vi "Buffered Stream to Tab-Delimited Text File.vi"() -> ()   [LabVIEW 2023]
doc: "Demonstrates the use of File I/O and Array functions to stream data to a tab-delimited text file. This example manages memory in an efficient manner to stream data to the text file at a high rate."
panel:
  out "Streaming Rate (MB/sec)":dbl
  # "Overview: Demonstrates the use of File I/O and Array functions to stream data to a tab-delimited text file. This example manages memory in an efficient manner to stream data to the text file at a high rate.\nInstructions:\n1. Run this VI, which streams data to a tab-delimited text file for 1 second.\n2. Open the [LabVIEW Data]\\Example Streamed Spreadsheet Data.txt file in a spreadsheet application, such as Microsoft Excel. The data in the file should automatically populate in the spreadsheet.\n3. Close the spreadsheet application.\n4. Delete the Example Streamed Spreadsheet Data.txt file after using this VI."
  # "Returns the rate at which LabVIEW streams data to a tab-delimited text file in megabytes per second."
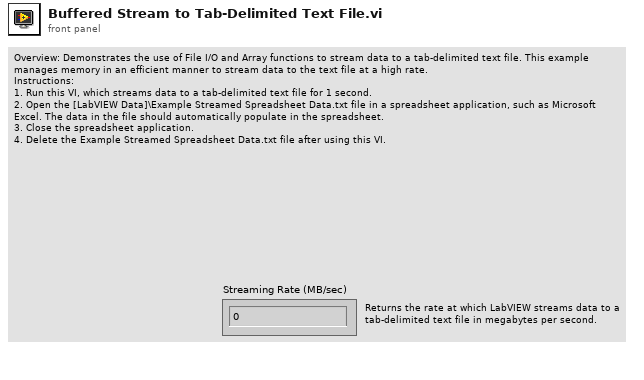
[diagram p1: front panel]
types:
  T1 = enum16{"open", "replace", "create", "open or create", "replace or create", "replace or create with confirmation"}
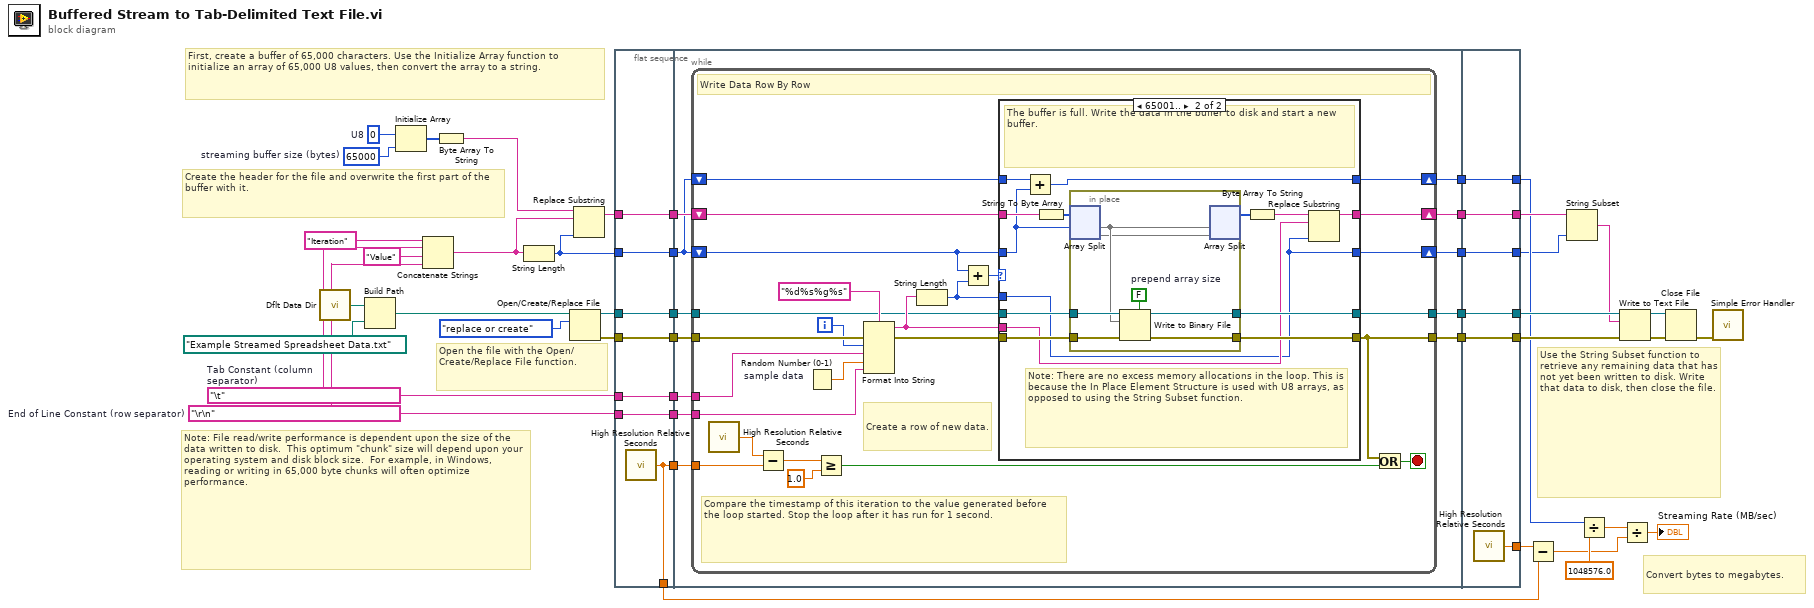
[diagram p0: block diagram]
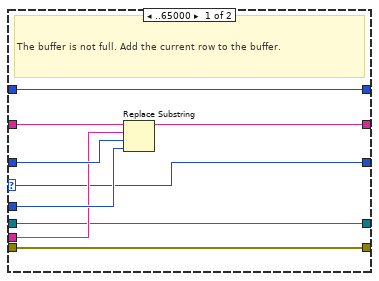
[diagram p2: hidden frame]
diagram:
  w27 = 65000  # streaming buffer size (bytes)
  w40 = u8 0  # U8
  w29 = "\r\n"  # End of Line Constant (row separator)
  w28 = "\t"  # Tab Constant (column separator)
  # "Open the file with the Open/Create/Replace File function."
  # "Create the header for the file and overwrite the first part of the buffer with it."
  # "First, create a buffer of 65,000 characters. Use the Initialize Array function to initialize an array of 65,000 U8 values, then convert the array to a string."
  # "Note: File read/write performance is dependent upon the size of the data written to disk.  This optimum \"chunk\" size will depend upon your operating system and disk block size.  For example, in Windows, reading or writing in 65,000 byte chunks will often optimize performance."
  # "Convert bytes to megabytes."
  # "Use the String Subset function to retrieve any remaining data that has not yet been written to disk. Write that data to disk, then close the file."
  n1 = call <vilib>:"Dflt Data Dir.vi"() -> ("App:Default Data Directory"=w24:path)
  n2 = Build Path(base path=w24, name or relative path=path "Example Streamed Spreadsheet Data.txt" ("default name")) -> (appended path=w23:path)
  n3 = Initialize Array(w40, w27) -> (w39:u8[])
  n4 = Concatenate Strings("Iteration", w28, "Value", w29) -> (w21:string)
  n5 = Byte Array To String(unsigned byte array=w39) -> (string=w37:string)
  n6 = String Length(string=w21) -> (length=w18:i32)
  n7 = Open/Create/Replace File(file path (use dialog)=w23, operation (0:open)=T1."replace or create") -> (refnum out=w41:refnum<file>, error out=w42:errorcluster)  [unwired: 4 in, 1 out]
  n8 = Replace Substring(2:w18, 4:w21, 5:w37) -> (1:w38:string)  [unwired: 1 in, 1 out]
  n9 = flat-sequence {
    tunnel: w18 -> [w46]
    tunnel: w28 -> [w47]
    tunnel: w29 -> [w48]
    tunnel: w38 -> [w49]
    tunnel: w41 -> [w50]
    tunnel: w42 -> [w51]
    tunnel: [w51] -> w17
    tunnel: [w50] -> w16
    tunnel: [w49] -> w15
    tunnel: [w48] -> w14
    tunnel: [w47] -> w13
    tunnel: [w45] -> w12
    tunnel: [w46] -> w11
    tunnel: [w45] -> w1
    tunnel: w17 -> [w63]
    tunnel: w16 -> [w62]
    tunnel: w15 -> [w61]
    tunnel: w14 -> [w57]
    tunnel: w13 -> [w56]
    tunnel: w12 -> [w52]
    tunnel: w11 -> [w53]
    tunnel: [w60] -> w10
    tunnel: [w59] -> w9
    tunnel: [w58] -> w8
    tunnel: [w55] -> w7
    tunnel: [w54] -> w6
    tunnel: [w120] -> w19
    tunnel: [w121] -> w20
    tunnel: [w122] -> w34
    tunnel: [w123] -> w35
    tunnel: [w124] -> w36
    tunnel: w10 -> [w124]
    tunnel: w9 -> [w123]
    tunnel: w8 -> [w122]
    tunnel: w7 -> [w121]
    tunnel: w6 -> [w120]
    tunnel: [w119] -> w5
    frame #0 {
      n10 = call <vilib>:"High Resolution Relative Seconds.vi"() -> ("relative seconds"=w45:dbl)
    }
    frame #1 {
      n11 = while {
        shift-right: [w79] -> w60
        shift-left: w61 -> [w82]
        shift-right: [w76] -> w54
        shift-left: w53 -> [w81]
        tunnel: w57 -> [w73]
        tunnel: w56 -> [w72]
        shift-right: [w69] -> w55
        shift-left: w53 -> [w70]
        tunnel: w52 -> [w68]
        tunnel: w63 -> [w88]
        tunnel: [w75] -> w59
        tunnel: w62 -> [w77]
        tunnel: [w78] -> w58
        i -> [w74]
        stop <- w85 stop-if-true
        # "Create a row of new data."
        # "Compare the timestamp of this iteration to the value generated before the loop started. Stop the loop after it has run for 1 second."
        # "Write Data Row By Row"
        n12 = call <vilib>:"High Resolution Relative Seconds.vi"() -> ("relative seconds"=w67:dbl)
        n13 = Subtract(x=w67, y=w68) -> (x-y=w66:dbl)
        n14 = Random Number (0-1) "sample data"() -> (number: 0 to 1=w71:dbl)
        n15 = Greater Or Equal?(x=w66, y=1.0) -> (x >= y?=w64:bool)
        n16 = Format Into String(format string="%d%s%g%s", error in=w88, w74, w72, w71, w73) -> (resulting string=w83:string, error out=w86:errorcluster)  [unwired: 1 in]
        n17 = String Length(string=w83) -> (length=w80:i32)
        n18 = Add(x=w81, y=w80) -> (x+y=w84:i32)
        n19 = case shown="65001.." w84 {
          selector: w84 -> [w90 _]
          tunnel: w86 -> [w92 w109]
          tunnel: w83 -> [w94 w102]
          tunnel: w82 -> [w97 w107]
          tunnel: w81 -> [w95 w98]
          tunnel: w80 -> [w96 w101]
          tunnel: [w93 w103] -> w79
          tunnel: [w92 w108] -> w75
          tunnel: [w91 w110] -> w78
          tunnel: w77 -> [w91 w111]
          tunnel: [w90 w101] -> w76
          tunnel: w70 -> [w89 w100]
          tunnel: [w89 w99] -> w69
          frame ..65000 {
            # "The buffer is not full. Add the current row to the buffer."
            n20 = Replace Substring(2:w96, 3:w95, 4:w94, 5:w97) -> (1:w93:string)  [unwired: 1 out]
          }
          frame 65001.. {
            # "Note: There are no excess memory allocations in the loop. This is because the In Place Element Structure is used with U8 arrays, as opposed to using the String Subset function."
            # "The buffer is full. Write the data in the buffer to disk and start a new buffer."
            n21 = Add(x=w100, y=w98) -> (x+y=w99:i32)
            n22 = String To Byte Array(string=w107) -> (unsigned byte array=w106:u8[])
            n23 = in-place {
              in-place-border: w111 -> [w118]
              in-place-border: [w117] -> w110
              in-place-border: w109 -> [w116]
              in-place-border: [w115] -> w108
              w112 = FALSE  # prepend array size
              n24 = in-place-split #1(w106, w98) -> (w114:u8[], w113:u8[])
              n25 = Write to Binary File(file (use dialog)=w118, data=w114, error in=w116, 5:w112) -> (refnum out=w117:refnum<file>, error out=w115:errorcluster)  [unwired: 2 in, 1 out]
              n26 = in-place-split #1(w114, w113) -> (w105:u8[])  [unwired: 1 out]
            }
            n27 = Byte Array To String(unsigned byte array=w105) -> (string=w104:string)
            n28 = Replace Substring(2:w101, 4:w102, 5:w104) -> (1:w103:string)  [unwired: 1 in, 1 out]
          }
        }
        n29 = Or(x=w75, y=w64) -> (x .or. y?=w85:bool)
      }
    }
    frame #2 {
      n30 = call <vilib>:"High Resolution Relative Seconds.vi"() -> ("relative seconds"=w119:dbl)
    }
  }
  n31 = Subtract(x=w5, y=w1) -> (x-y=w3:dbl)
  n32 = String Subset(string=w36, length (rest)=w19) -> (substring=w33:string)  [unwired: 1 in]
  n33 = Divide(x=w20, y=1048576.0) -> (x/y=w4:dbl)
  n34 = Write to Text File(file (use dialog)=w34, text=w33, error in=w35) -> (refnum out=w31:refnum<file>, error out=w32:errorcluster)  [unwired: 1 in, 1 out]
  n35 = Divide(x=w4, y=w3) -> (x/y=→"Streaming Rate (MB/sec)":dbl)
  n36 = Close File(refnum=w31, error in=w32) -> (error out=w30:errorcluster)  [unwired: 1 out]
  n37 = call <vilib>:"Simple Error Handler.vi"("error in (no error)"=w30) -> ()  [unwired: 4 in, 5 out]
